vi "EVALSHA.vi"(0 "TCP session in":refnum<k5>, 5 "script SHA":string, 7 "KEYS":string[](array[string]), 9 "ARGV":string[](array[string]), 11 "error in":errorcluster) -> (4 "TCP session out":refnum<k5>, 6 "Data":T1, 8 "string data":string[](array[string]), 15 "error out":errorcluster)   [LabVIEW 2023]
uses:
  SubVIs/Controls/redis-data.ctl
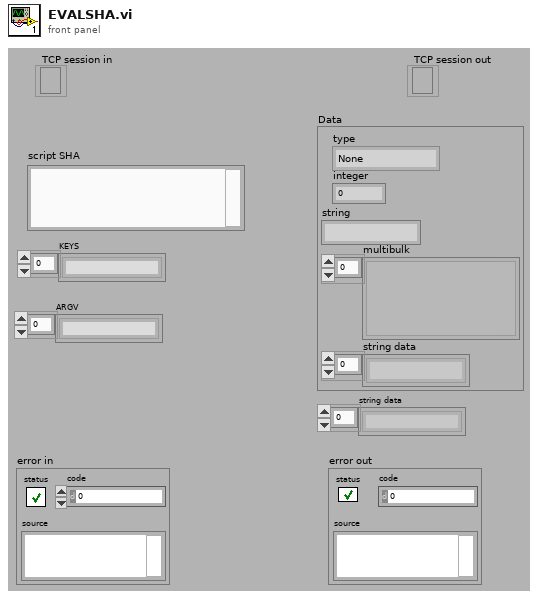
[diagram p1: front panel]
types:
  T1 = typedef "redis-data.ctl" = cluster{"type":enum16{"None", "Error", "Status", "Nil", "Integer", "String", "Multibulk"}, "integer":i64, "string":string, "multibulk":variant[], "string data":string[]}
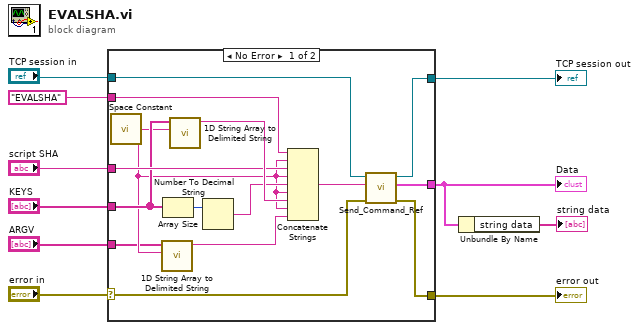
[diagram p0: block diagram]
diagram:
  n1 = case shown="No Error" "error in" {
    selector: "error in" -> [w25 w27]
    tunnel: "script SHA" -> [w15 _]
    tunnel: "EVALSHA" -> [w16 _]
    tunnel: "TCP session in" -> [w22 w26]
    tunnel: [w24 w27] -> w8
    tunnel: [w23 _] -> w1
    tunnel: [w21 w26] -> w5
    tunnel: "KEYS" -> [w14 _]
    tunnel: "ARGV" -> [w12 _]
    frame No Error {
      n2 = call <vilib>:"Space Constant.vi"() -> ("String"=w13:string)
      n3 = call <vilib>:"1D String Array to Delimited String.vi"("delimiter"=w13, "string array"=w12) -> ("delimited string"=w11:string)  [unwired: 9 in]
      n4 = Array Size(array=w14) -> (size(s)=w18:i32)
      n5 = call <vilib>:"1D String Array to Delimited String.vi"("delimiter"=w13, "string array"=w14) -> ("delimited string"=w20:string)  [unwired: 9 in]
      n6 = Number To Decimal String(number=w18) -> (decimal integer string=w19:string)  [unwired: 1 in]
      n7 = Concatenate Strings(w16, w13, w15, w13, w19, w13, w20, w13, w11) -> (w17:string)
      n8 = call "Send_Command_Ref.vi"("error in"=w25, "command"=w17, "TCP session in"=w22) -> ("error out"=w24:errorcluster, "Data"=w23:T1, "TCP session out"=w21:refnum<k5>)  [unwired: 6 in]
    }
    frame Error {
    }
  }
  "error out" <- w8
  "TCP session out" <- w5
  "Data" <- w1
  n9 = Unbundle By Name(w1) -> ("string data"=→"string data":string[])
